vi "prepareToNoAck.vi"(6 "iteration":i32, 7 "cmdLost":bool, 8 "error in (no error)":errorcluster, 9 "lostCmdId":i32, 10 "cmd":string, 11 "TcpServer in":refnum<class "TcpServer.lvclass">) -> (0 "error out":errorcluster, 2 "JSON string":string, 3 "TcpServer out":refnum<class "TcpServer.lvclass">)   [LabVIEW 2018, in "TcpServer.lvclass"]
doc: "Prepare the command received to send the noAck to TCP Client."
uses:
  TcpServer.lvclass
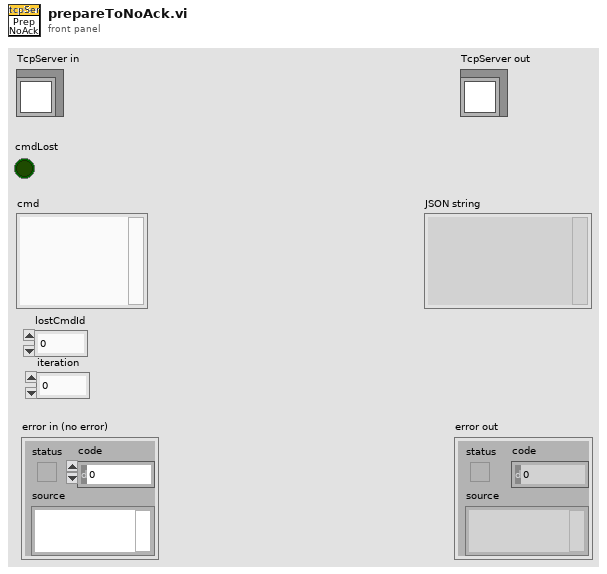
[diagram p1: front panel]
types:
  T1 = cluster{"cmdName":string, "cmdId":i32, "cmdStatus":string}
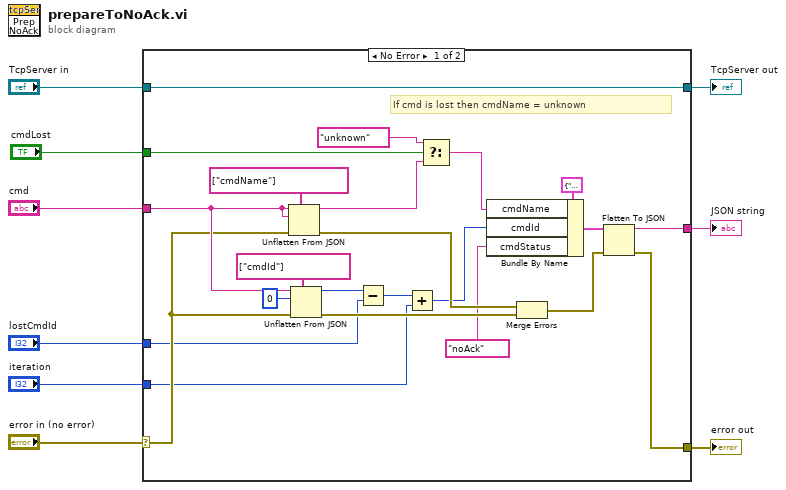
[diagram p0: block diagram]
diagram:
  n1 = case shown="No Error" "error in (no error)" {
    selector: "error in (no error)" -> [w24 w34]
    tunnel: [w20 w34] -> w8
    tunnel: [w32 w33] -> w6
    tunnel: "TcpServer in" -> [w32 w33]
    tunnel: "cmd" -> [w29 _]
    tunnel: [w25 _] -> w4
    tunnel: "lostCmdId" -> [w16 _]
    tunnel: "iteration" -> [w18 _]
    tunnel: "cmdLost" -> [w13 _]
    frame No Error {
      # "If cmd is lost then cmdName = unknown"
      n2 = Unflatten From JSON(path=string[] ["cmdName"], JSON string=w29, type and defaults=w29, error in (no error)=w24) -> (value=w11:string, error out=w23:errorcluster)  [unwired: 3 in]
      n3 = Unflatten From JSON(path=string[] ["cmdId"], JSON string=w29, type and defaults=0, error in (no error)=w24) -> (value=w17:i32, error out=w22:errorcluster)  [unwired: 3 in]
      n4 = Subtract(x=w17, y=w16) -> (x-y=w15:i32)
      n5 = Add(x=w15, y=w18) -> (x+y=w19:i32)
      n6 = Select(t="unknown", s=w13, f=w11) -> (s? t:f=w10:string)
      n7 = Bundle By Name(cluster=T1 {"cmdName"="", "cmdId"=0, "cmdStatus"=""}, "cmdName"=w10, "cmdId"=w19, "cmdStatus"="noAck") -> (w26:T1)
      n8 = Merge Errors(w23, w22) -> (w21:errorcluster)
      n9 = Flatten To JSON(anything=w26, error in (no error)=w21) -> (JSON string=w25:string, 11:w20:errorcluster)  [unwired: 1 in]
    }
    frame Error {
    }
  }
  "error out" <- w8
  "TcpServer out" <- w6
  "JSON string" <- w4
